vi "VI Scripting with Structures - Timed Sequence.vi"   [LabVIEW 2023]
doc: "This example contains sample code demonstrating common VI Scripting navigational tasks relating to Timed Sequences."
panel:
  # "Overview: Illustrates several TimedSequence properties and methods used for inspecting and modifying Timed Sequences with VI Scripting.\nInstructions:\nOpen the block diagram of this VI to see several examples of properties and methods related to Timed Sequences and VI Scripting.\n\nNote: Browse the diagram of this example to learn about VI Scripting concepts. This example is not meant to be run."
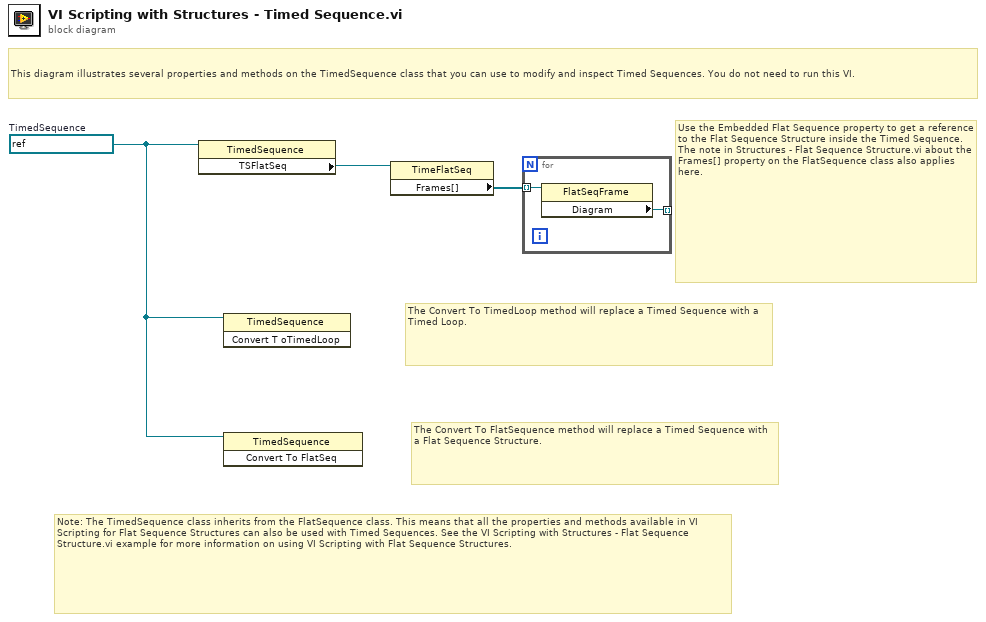
[diagram p0: block diagram]
diagram:
  w3 = refnum<vi> refnum  # TimedSequence
  # "Note: The TimedSequence class inherits from the FlatSequence class. This means that all the properties and methods available in VI Scripting for Flat Sequence Structures can also be used with Timed Sequences. See the VI Scripting with Structures - Flat Sequence Structure.vi example for more information on using VI Scripting with Flat Sequence Structures."
  # "The Convert To FlatSequence method will replace a Timed Sequence with a Flat Sequence Structure."
  # "The Convert To TimedLoop method will replace a Timed Sequence with a Timed Loop."
  # "Use the Embedded Flat Sequence property to get a reference to the Flat Sequence Structure inside the Timed Sequence. The note in Structures - Flat Sequence Structure.vi about the Frames[] property on the FlatSequence class also applies here."
  # "This diagram illustrates several properties and methods on the TimedSequence class that you can use to modify and inspect Timed Sequences. You do not need to run this VI."
  n1 = property class="TimedSequence"(reference=w3) -> ("TSFlatSeq"=w2:refnum<vi>)  [unwired: 1 in, 2 out]
  n2 = invoke class="TimedSequence" method="Convert T oTimedLoop"(reference=w3) -> ()  [unwired: 2 in, 3 out]
  n3 = invoke class="TimedSequence" method="Convert To FlatSeq"(reference=w3) -> ()  [unwired: 2 in, 3 out]
  n4 = property class="TimeFlatSeq"(reference=w2) -> ("Frames[]"=w1:refnum<vi>[])  [unwired: 1 in, 2 out]
  n5 = for {
    tunnel: w1 -> [w5] mode=indexing
    tunnel: [w4] -> _ mode=indexing
    n6 = property class="FlatSeqFrame"(reference=w5) -> ("Diagram"=w4:refnum<vi>)  [unwired: 1 in, 2 out]
  }
